vi "Open by Index.vi"(7 "Enable Events (T)":bool=TRUE, 8 "Error In":errorcluster, 11 "Device Index":i32) -> (0 "Error Out":errorcluster, 2 "Event Refnum":refnum<event-registration>, 3 "Xbox One Controller Ref":T1)   [LabVIEW 2021, in "LMH-Xbox-One-Controller.lvlib"]
doc: "Open a connection to an Xbox One Controller."
uses:
  <instrlib>/Xbox-One-Controller/LMH-Xbox-One-Controller.lvlib
  <instrlib>/Xbox-One-Controller/Private/Type Defs/Xbox One Controller Ref.ctl
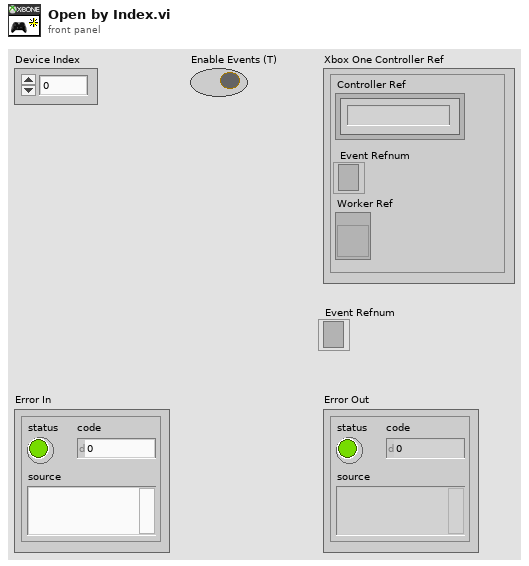
[diagram p1: front panel]
types:
  T1 = typedef "LMH-Xbox-One-Controller.lvlib/Xbox One Controller Ref.ctl" = cluster{"Controller Ref":refnum<k1>, "Event Refnum":refnum<event-registration>, "Worker Ref":refnum<vi>}
  T2 = typedef "LMH-Xbox-One-Controller.lvlib/Events.ctl" = cluster{"A":refnum<user-event>, "B":refnum<user-event>, "X":refnum<user-event>, "Y":refnum<user-event>, "Left Bumper":refnum<user-event>, "Right Bumper":refnum<user-event>, "View":refnum<user-event>, "Menu":refnum<user-event>, "Left Stick":refnum<user-event>, "Right Stick":refnum<user-event>}
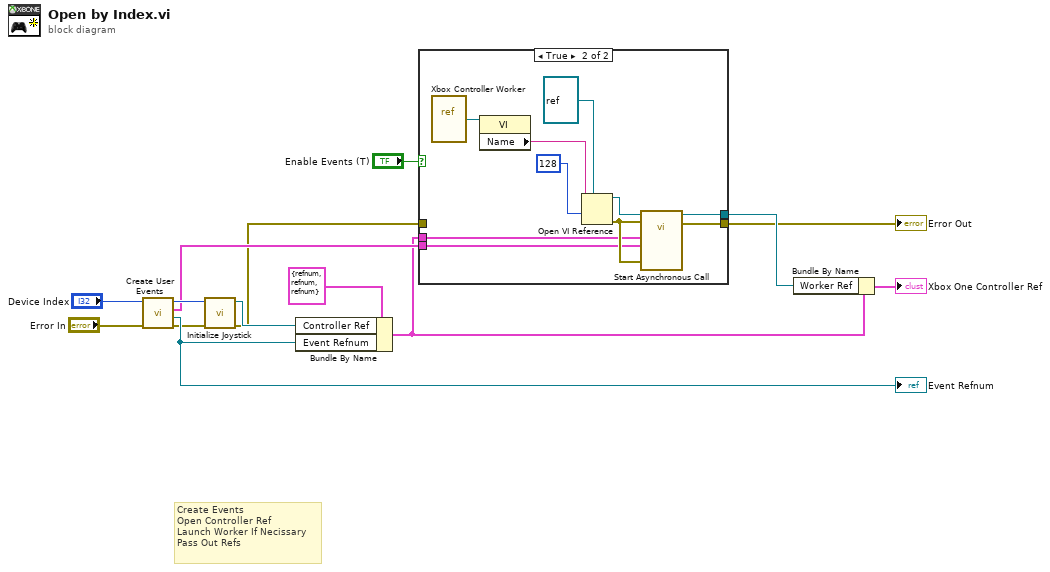
[diagram p0: block diagram]
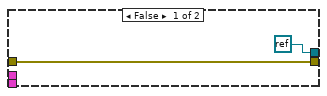
[diagram p2: hidden frame]
diagram:
  # "Create Events\nOpen Controller Ref\nLaunch Worker If Necissary\nPass Out Refs"
  n1 = call <instrlib>:"Create User Events.vi"("Error In"="Error In") -> ("Error Out"=w6:errorcluster, "Event Refnum"=w7:refnum<event-registration>, "Events"=w11:T2)  [unwired: 8 in]
  "Event Refnum" <- w7
  n2 = call <vilib>:"Initialize Joystick.vi"("error in (no error)"=w6, "device index"="Device Index") -> ("error out"=w4:errorcluster, "device ID"=w5:refnum<k1>)  [unwired: 8 in]
  n3 = Bundle By Name(cluster=T1 {"Controller Ref"=refnum, "Event Refnum"=refnum, "Worker Ref"=refnum} ("Xbox One Controller Ref"), "Controller Ref"=w5, "Event Refnum"=w7) -> (w8:T1)
  n4 = case shown="True" "Enable Events (T)" {
    tunnel: w11 -> [_ w19]
    tunnel: [refnum<k0> refnum w18] -> w9
    tunnel: w8 -> [_ w17]
    tunnel: [w14 w16] -> w3
    tunnel: w4 -> [w14 _]
    frame False {
    }
    frame True {
      n5 = vi-ref <instrlib>:"Xbox Controller Worker.vi"() -> (w25:refnum<vi>)
      n6 = property class="VI"(reference=w25) -> ("Name"=w21:string)  [unwired: 1 in, 2 out]
      n7 = Open VI Reference(type specifier VI Refnum (for type only)=refnum<vi> refnum, vi path=w21, options=128) -> (vi reference=w22:refnum<vi>, error out=w20:errorcluster)  [unwired: 3 in]
      n8 = call-by-ref "Start Asynchronous Call"(reference=w22, error in=w20, "Error In"=w20, "Events"=w19, "Xbox One Controller Ref"=w17) -> (reference out=w18:refnum<vi>, error out=w16:errorcluster)  [unwired: 8 in, 1 out]
    }
  }
  "Error Out" <- w3
  n9 = Bundle By Name(cluster=w8, "Worker Ref"=w9) -> (→"Xbox One Controller Ref":T1)
